vi "CCSTiming.vi"(7 "FileTimestamp":timestamp, 11 "array":string[](array[string])) -> (2 "extended precision float":ext format="%.6f", 3 "timestamp out":timestamp format="%^<%.3X\n%x>T")   [LabVIEW 2014]
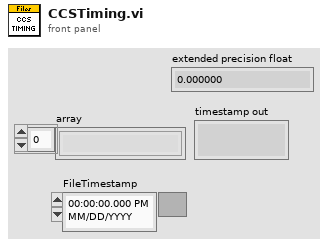
[diagram p1: front panel]
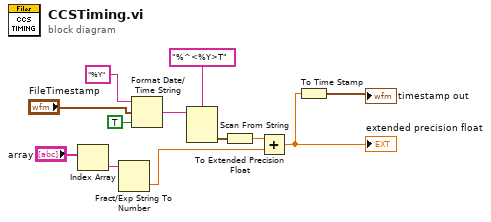
[diagram p0: block diagram]
diagram:
  n1 = Index Array(array="array") -> (element=w8:string)  [unwired: 1 in]
  n2 = Fract/Exp String To Number(string=w8) -> (number=w3:dbl)  [unwired: 3 in, 1 out]
  n3 = Format Date/Time String(time format string (%c)="%Y", seconds (now)="FileTimestamp", UTC format=TRUE) -> (date/time string=w7:string)
  n4 = Scan From String(format string="%^<%Y>T", input string=w7) -> (output 1=w5:timestamp)  [unwired: 3 in, 3 out]
  n5 = To Extended Precision Float(1:w5) -> (0:w4:ext)
  n6 = Add(x=w4, y=w3) -> (x+y=w2:ext)
  "extended precision float" <- w2
  n7 = To Time Stamp(1:w2) -> (0:→"timestamp out":timestamp)
